vi "ZERO tool variable.vi"(8 "error in (no error)":errorcluster, 11 "Var index":i32[](array[numeric])) -> (0 "error out":errorcluster)   [LabVIEW 2011]
doc: "This VI calculates a new offset for a list of tool variables. It assumes that the physical quantity that is currently being measured is zero. The new scaling coefficients for the variable is written to the Variables.ini file."
uses:
  Common/Variable List Common Analog.ctl
  Tool/Variable List Tool Analog.ctl
  Action Analog Handler.ctl
  emi Lib/Basic/0 - General/App/emi_Application Folder.vi
  <vilib>/Utility/VariantDataType/GetNumericInfo.vi
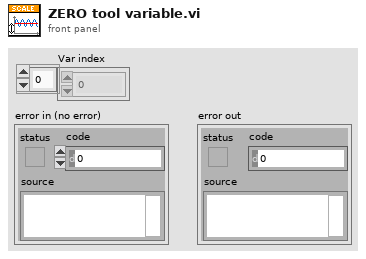
[diagram p1: front panel]
types:
  T1 = typedef "Variable List Tool Analog.ctl" = enum16{"Tool Max Temperature", "Tool (Controller) Temperature", "Tool Supply Voltage", "Tool (Controller) Current", "Tool Acceleration X", "Tool Acceleration Y", "Tool Acceleration Z", "Tool Acceleration Sum", "Tool Inclination", "Tool Rotation", "Tool GP Sensor 1", "Tool GP Sensor 2", "Tool (Pressure 1) Temperature", "Tool Pressure 1 RAW", "Tool (Pressure 2) Temperature", "Tool Pressure 2 RAW", "Tool (Solenoid) Temperature", "Tool Solenoid Position", "PSU Temp", "Head Voltage", "PSU Main Voltage out", "PSU Main Current out", "Upper Tension Sub Temp", "Tool Upper Tension Sub Raw", "Lower Tension Sub Temp", "Tool Lower Tension Sub Raw", "Tool Var27 - Reserved", "Tool Var28 - Reserved", "Tool Var29 - Reserved", "Tool Var30 - Reserved", "Stroke Extension", "Stroke In Force", "Stroke Out Force", "Stroke Force", "Stroker Pressure 1", "Stroker Pressure 2", "Stroker Upper Tension Sub", "Stroker Lower Tension Sub", "Stroker Var09 - Reserved", "Stroker Var10 - Reserved", "Tractor Upper Tension Sub", "Tractor Lower Tension Sub", "Tractor Var03 - Reserved", "Tractor Var04 - Reserved", "Tool Temperature sensor", "Tool Motor Voltage", "Tool Motor Current", "Tool Motor Torque", "Tool weight on bit", "Tool Motor RPM"}
  T2 = typedef "Variable List Common Analog.ctl" = enum16{"HVPSU Head Voltage", "HVPSU TS Voltage", "HVPSU Current", "PCP Cable Resistance", "Winch Depth", "Winch Line Speed", "Winch Wire Tension"}
  T3 = typedef "User Setting Analog Channel Bg.ctl" = cluster{"Scaling":T4, "Limits and responces":T5, "Allow Graph selection by user":bool, "Unit":u16}
  T4 = typedef "Scaling.ctl" = cluster{"Gain":dbl, "Offset":dbl}
  T5 = typedef "Alarm Setup Analog.ctl" = cluster{"Technical Error(NA)":T6, "LL":T6, "L":T6, "H":T6, "HH":T6, "Limits":T8}
  T6 = typedef "Alarm Responce.ctl" = cluster{"Action":T7, "Alarm":bool}
  T7 = typedef "Action List.ctl" = enum16{"No Action", "Stop Motor", "Turn Off HV"}
  T8 = typedef "Limits.ctl" = cluster{"LL":dbl, "L":dbl, "H":dbl, "HH":dbl}
  T9 = typedef "User Setting DigitalChannel.ctl" = cluster{"Responses":cluster{"Technical Error (NA)":T6, "OFF / FALSE":T10, "ON / TRUE":T10}}
  T10 = typedef "Alarm Responce dig.ctl" = cluster{"Action":T7, "Alarm":bool, "Exclamation":bool}
  T11 = typedef "Action Analog Handler.ctl" = enum16{"GET value", "GET Single Frequenzy", "GET All Values", "GET Waveform", "Get Numb Var", "SET Value", "START Buffer", "REG Variable", "BUF size(total antal sekund)", "PULS", "Get a Value at time", "Set initial waveform"}
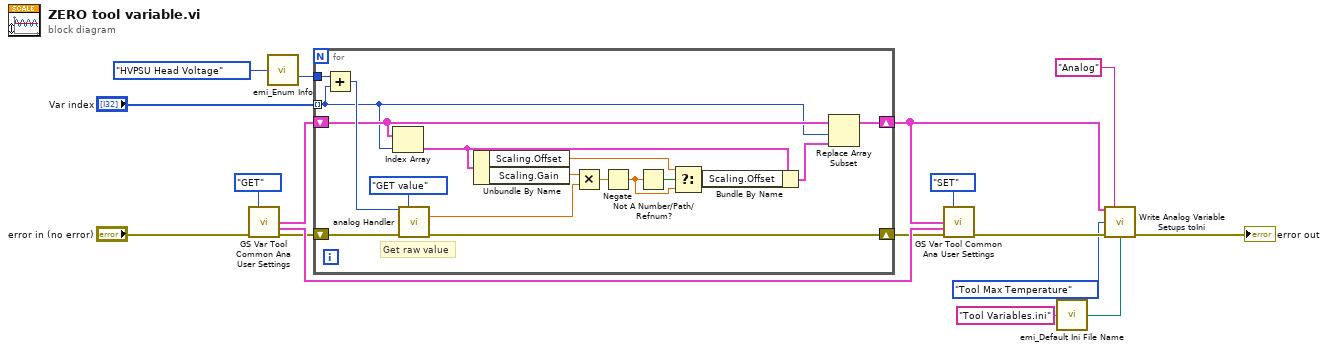
[diagram p0: block diagram]
diagram:
  n1 = call "GS Var Tool Common Ana User Settings.vi"("Action(GET)"=enum16{"GET", "SET"}."GET", "error in (no error)"="error in (no error)") -> ("Tool Analog var User settigns out"=w5:T3[], "Tool digital var User settigns out"=w8:T9[], "error out"=w3:errorcluster)  [unwired: 11 in]
  n2 = call "emi_Enum Info.vi"("Enum"=Variable_List_Common_Analog."HVPSU Head Voltage" ("First part list")) -> ("Numb Elements"=w4:i32)  [unwired: 11 in, 3 out]
  n3 = for {
    tunnel: "Var index" -> [w23] mode=indexing
    tunnel: w4 -> [w33]
    shift-right: [w24] -> w17
    shift-left: w5 -> [w26]
    shift-right: [w18] -> w7
    shift-left: w3 -> [w31]
    # "Get raw value"
    n4 = Add(x=w33, y=w23) -> (x+y=w32:i32)
    n5 = Index Array(array=w26, index=w23) -> (element=w27:T3)
    n6 = call "analog Handler.vi"("Variable Index"=w32, "Action"=Action_Analog_Handler."GET value" ("Action(GET)"), "error in (no error)"=w31) -> ("Value out"=w29:dbl, "error out"=w18:errorcluster)  [unwired: 7 in, 4 out]
    n7 = Unbundle By Name(w27) -> ("Scaling.Offset"=w21:dbl, "Scaling.Gain"=w30:dbl)
    n8 = Multiply(x=w30, y=w29) -> (x*y=w28:dbl)
    n9 = Negate(x=w28) -> (-x=w19:dbl)
    n10 = Not A Number/Path/Refnum?(number/path/refnum=w19) -> (NaN/Path/Refnum?=w22:bool)
    n11 = Select(t=w21, s=w22, f=w19) -> (s? t:f=w20:dbl)
    n12 = Bundle By Name(cluster=w27, "Scaling.Offset"=w20) -> (w25:T3)
    n13 = Replace Array Subset(array=w26, new element=w25, index=w23) -> (w24:T3[])
  }
  n14 = call "GS Var Tool Common Ana User Settings.vi"("Action(GET)"=enum16{"GET", "SET"}."SET", "Tool analog var User settigns in"=w17, "Tool digital var User settigns in"=w8, "error in (no error)"=w7) -> ("error out"=w15:errorcluster)  [unwired: 9 in, 2 out]
  n15 = call "emi_Default Ini File Name.vi"("Name"="Tool Variables.ini" ("name or relative path")) -> ("Path"=w12:path)  [unwired: 13 in, 1 out]
  n16 = call "Write Analog Variable Setups toIni.vi"("error in (no error)"=w15, "Path"=w12, "Enum with Variable List"=Variable_List_Tool_Analog."Tool Max Temperature" ("Variable ID"), "Analog User settigns"=w17, "Section(\"Default\")"="Analog" ("Section(\"Default\")")) -> ("error out"=→"error out":errorcluster)  [unwired: 10 in]
